vi "eGateHSP_StopConfiguration.vi"(8 "Fehler (Eingang, kein Fehler)":errorcluster) -> (0 "Fehler (Ausgang)":errorcluster)   [LabVIEW 2016]
uses:
  eGateHighSpeedPort.dll
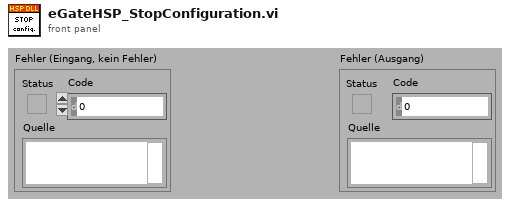
[diagram p1: front panel]
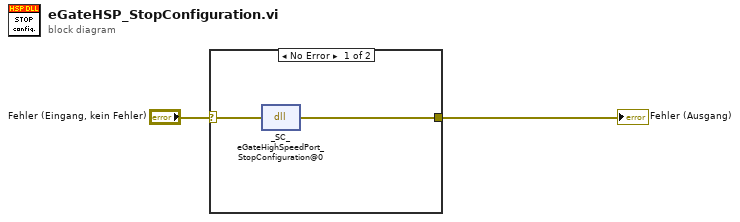
[diagram p0: block diagram]
diagram:
  n1 = case shown="No Error" "Fehler (Eingang, kein Fehler)" {
    selector: "Fehler (Eingang, kein Fehler)" -> [w4 _]
    tunnel: [w3 _] -> w1
    frame No Error {
      n2 = dll-call lib="eGateHighSpeedPort.dll" fn="_SC_eGateHighSpeedPort_StopConfiguration@0"(error in=w4) -> (error out=w3:errorcluster)  [unwired: 3 in, 1 out]
    }
    frame Error {
    }
  }
  "Fehler (Ausgang)" <- w1
